vi "Power Measurement Error Codes.vi"(7 "Detector Type (RMS)":i32(ring) items=["RMS", "Minimum", "Maximum"], 8 "error in (no error)":errorcluster, 9 "Result Type (Current)":i32(ring) items=["Current", "Average", "Peak"], 10 "Instance (1)":i32=1, 11 "VISA resource name":refnum<visa-resource-name>) -> (0 "error out":errorcluster, 1 "Error Codes":i32[](array[numeric]), 2 "Reliability":i32, 3 "VISA resource name out":refnum<visa-resource-name>)   [LabVIEW 2015, in "Rohde&Schwarz CMXP GPRF.lvlib"]
doc: "Returns a single-value error code for each result.\n\nAttribute:\nRSCMXPGPRF_ATTR_POWER_MEASUREMENT_POWER_CURRENT\nRSCMXPGPRF_ATTR_POWER_MEASUREMENT_LIMIT_CHECK_RESULT_MINIMUM_CURRENT\nRSCMXPGPRF_ATTR_POWER_MEASUREMENT_LIMIT_CHECK_RESULT_MAXIMUM_CURRENT\nRSCMXPGPRF_ATTR_POWER_MEASUREMENT_LIMIT_CHECK_RESULT_AVERAGE\nRSCMXPGPRF_ATTR_POWER_MEASUREMENT_LIMIT_CHECK_RESULT_PEAK_MINIMUM\nRSCMXPGPRF_ATTR_POWER_MEASUREMENT_LIMIT_CHECK_RESULT_PEAK_MAXIMUM\n\nRemote-control commands:\nCALCulate:GPRF:MEAS<i>:POWer:RMS:CURRent?\nCALCulate:GPRF:MEAS<i>:POWer:MINimum:CURRent?\nCALCulate:GPRF:MEAS<i>:POWer:MAXimum:CURRent?\nCALCulate:GPRF:MEAS<i>:POWer:AVERage?\nCALCulate:GPRF:MEAS<i>:POWer:PEAK:MINimum?\nCALCulate:GPRF:MEAS<i>:POWer:PEAK:MAXimum?"
uses:
  <instrlib>/Rohde&Schwarz CMXP GPRF/Rohde&Schwarz CMXP GPRF.lvlib
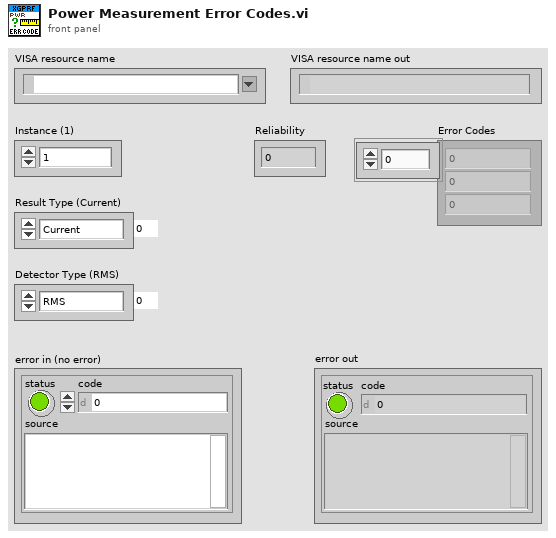
[diagram p1: front panel]
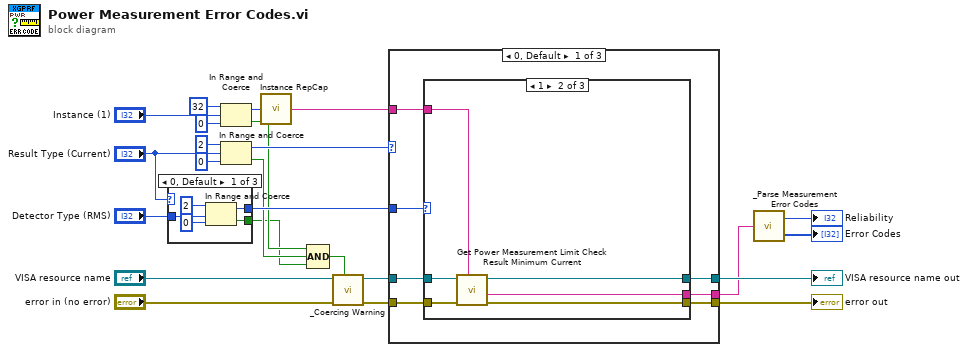
[diagram p0: block diagram]
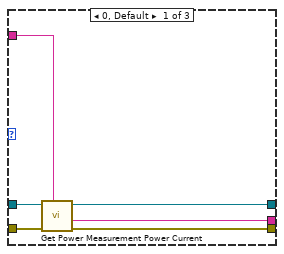
[diagram p2: hidden frame]
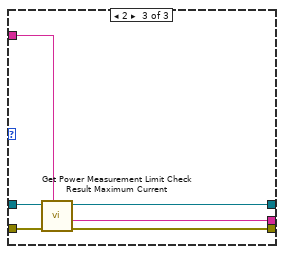
[diagram p3: hidden frame]
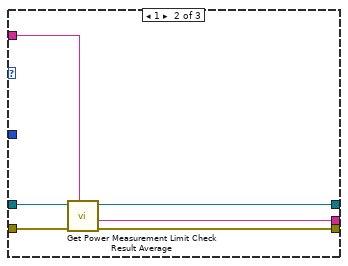
[diagram p4: hidden frame]
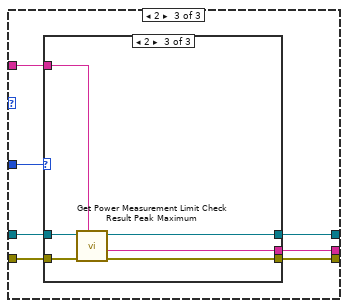
[diagram p5: hidden frame]
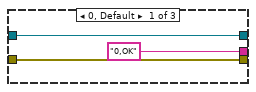
[diagram p6: hidden frame]
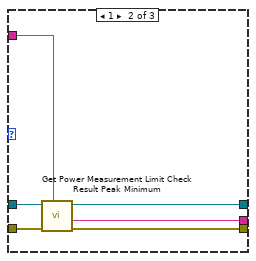
[diagram p7: hidden frame]
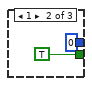
[diagram p8: hidden frame]
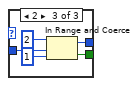
[diagram p9: hidden frame]
diagram:
  n1 = case shown="0, Default" "Result Type (Current)" {
    tunnel: [w28 TRUE w35] -> w2
    tunnel: [w27 0 ("upper limit") w34] -> w7
    tunnel: "Detector Type (RMS)" -> [w26 _ w33]
    frame 0, Default {
      n2 = In Range and Coerce(upper limit=2, x=w26, lower limit=0) -> (coerced(x)=w27:i32, In Range?=w28:bool)
    }
    frame 1 {
    }
    frame 2 {
      n3 = In Range and Coerce(upper limit=2, x=w33, lower limit=1) -> (coerced(x)=w34:i32, In Range?=w35:bool)
    }
  }
  n4 = In Range and Coerce(upper limit=32, x="Instance (1)", lower limit=0) -> (coerced(x)=w14:i32, In Range?=w3:bool)
  n5 = In Range and Coerce(upper limit=2, x="Result Type (Current)", lower limit=0) -> (coerced(x)=w8:i32, In Range?=w4:bool)
  n6 = call <instrlib>:"Instance RepCap.vi"("instance  in"=w14) -> ("instance out"=w9:string)
  n7 = Compound Arithmetic op=AND(w3, w4, w2) -> (w22:bool)
  n8 = call <instrlib>:"_Coercing Warning.vi"("In Range?"=w22, "error in (no error)"="error in (no error)", "VISA resource name"="VISA resource name") -> ("error out"=w13:errorcluster, "VISA resource name out"=w12:refnum<visa-resource-name>)  [unwired: 7 in]
  n9 = case shown="0, Default" w8 {
    tunnel: w13 -> [w43 w67 w74]
    tunnel: w12 -> [w42 w66 w73]
    tunnel: [w38 w63 w69] -> w11
    tunnel: [w37 w62 w68] -> w10
    tunnel: w7 -> [w41 _ w72]
    tunnel: [w40 w65 w71] -> w1
    tunnel: w9 -> [w39 w64 w70]
    frame 0, Default {
      n10 = case shown="1" w41 {
        tunnel: w43 -> [w49 w55 w61]
        tunnel: w42 -> [w48 w54 w60]
        tunnel: [w45 w51 w57] -> w38
        tunnel: [w44 w50 w56] -> w37
        tunnel: [w47 w53 w59] -> w40
        tunnel: w39 -> [w46 w52 w58]
        frame 0, Default {
          n11 = call "Get Power Measurement Power Current"("Repeated Capabilities"=w46, "error in (no error)"=w49, "instrument handle"=w48) -> ("error out"=w45:errorcluster, "Power Measurement Power Current"=w47:string, "instrument handle out"=w44:refnum<visa-resource-name>)  [unwired: 6 in]
        }
        frame 1 {
          n12 = call "Get Power Measurement Limit Check Result Minimum Current"("Repeated Capabilities"=w52, "error in (no error)"=w55, "instrument handle"=w54) -> ("error out"=w51:errorcluster, "Power Measurement Limit Check Result Minimum Current"=w53:string, "instrument handle out"=w50:refnum<visa-resource-name>)  [unwired: 6 in]
        }
        frame 2 {
          n13 = call "Get Power Measurement Limit Check Result Maximum Current"("Repeated Capabilities"=w58, "error in (no error)"=w61, "instrument handle"=w60) -> ("error out"=w57:errorcluster, "Power Measurement Limit Check Result Maximum Current"=w59:string, "instrument handle out"=w56:refnum<visa-resource-name>)  [unwired: 6 in]
        }
      }
    }
    frame 1 {
      n14 = call "Get Power Measurement Limit Check Result Average"("Repeated Capabilities"=w64, "error in (no error)"=w67, "instrument handle"=w66) -> ("error out"=w63:errorcluster, "Power Measurement Limit Check Result Average"=w65:string, "instrument handle out"=w62:refnum<visa-resource-name>)  [unwired: 6 in]
    }
    frame 2 {
      n15 = case shown="2" w72 {
        tunnel: w74 -> [w76 w83 w89]
        tunnel: w73 -> [w75 w82 w88]
        tunnel: [w76 w79 w85] -> w69
        tunnel: [w75 w78 w84] -> w68
        tunnel: ["0,OK" ("Read Power Measurement Maximum Current") w81 w87] -> w71
        tunnel: w70 -> [_ w80 w86]
        frame 0, Default {
        }
        frame 1 {
          n16 = call "Get Power Measurement Limit Check Result Peak Minimum"("Repeated Capabilities"=w80, "error in (no error)"=w83, "instrument handle"=w82) -> ("error out"=w79:errorcluster, "Power Measurement Limit Check Result Peak Minimum"=w81:string, "instrument handle out"=w78:refnum<visa-resource-name>)  [unwired: 6 in]
        }
        frame 2 {
          n17 = call "Get Power Measurement Limit Check Result Peak Maximum"("Repeated Capabilities"=w86, "error in (no error)"=w89, "instrument handle"=w88) -> ("error out"=w85:errorcluster, "Power Measurement Limit Check Result Peak Maximum"=w87:string, "instrument handle out"=w84:refnum<visa-resource-name>)  [unwired: 6 in]
        }
      }
    }
  }
  "error out" <- w11
  "VISA resource name out" <- w10
  n18 = call <instrlib>:"_Parse Measurement Error Codes.vi"("String In"=w1) -> ("Reliability"=→"Reliability":i32, "Results"=→"Error Codes":i32[])
